vi "XNET Convert (Byte Array to Frame FlexRay).vi"(0 "session in":refnum<k21>, 5 "signal data":u8[](array[numeric]), 11 "error in (no error)":errorcluster) -> (4 "session out":refnum<k21>, 6 "frame data":T1[](array[typedef]) {"payload" format="%x"; "timestamp" format="%<%.7X\n%x>T"; "type" items=["FlexRay Data"=32, "FlexRay Null"=33, "FlexRay Symbol"=34, "Log Trigger"=225, "Start Trigger"=226]; "cycle count" max=63 step=1}, 14 "unused payloads":cluster{"payload":u8[]}[](array[cluster]), 15 "error out":errorcluster)   [LabVIEW 2018]
doc: "Converts signal data to NI-XNET FlexRay frame data."
uses:
  XNET Frame FlexRay.ctl
  XNET Frame Type FlexRay.ctl
  nixlvapi.dll
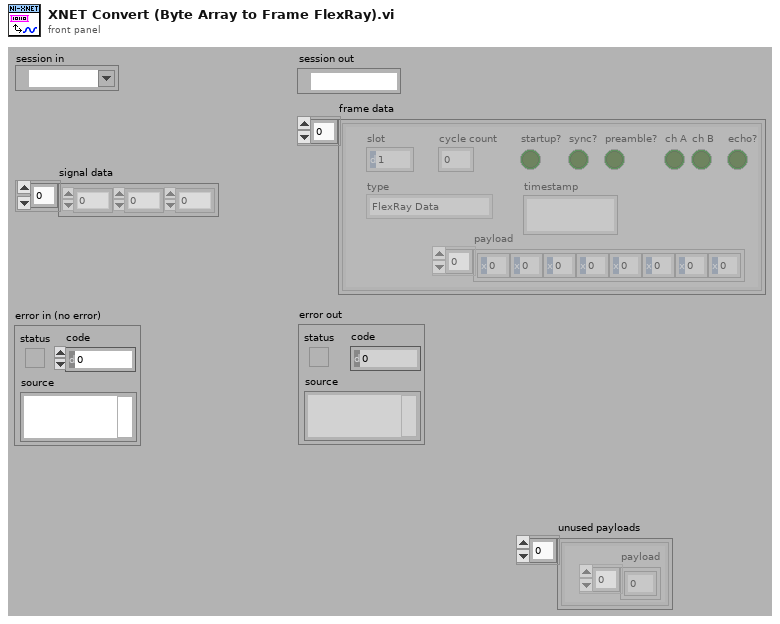
[diagram p1: front panel]
types:
  T1 = typedef "XNET Frame FlexRay.ctl" = cluster{"timestamp":timestamp, "payload":u8[], "slot":u16, "type":T2, "cycle count":u8, "startup?":bool, "sync?":bool, "preamble?":bool, "ch A":bool, "ch B":bool, "echo?":bool}
  T2 = typedef "XNET Frame Type FlexRay.ctl" = u8
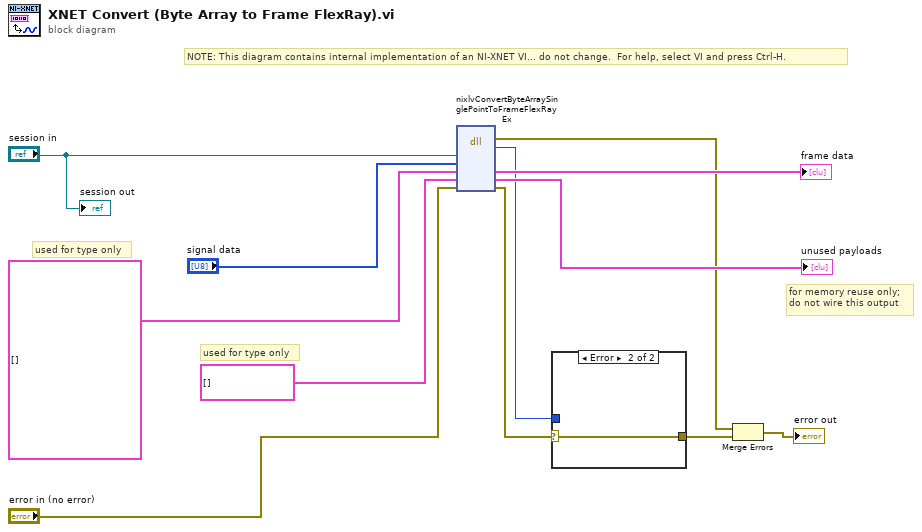
[diagram p0: block diagram]
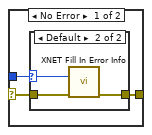
[diagram p2: hidden frame]
diagram:
  # "used for type only"
  # "for memory reuse only;\ndo not wire this output"
  # "used for type only"
  # "NOTE: This diagram contains internal implementation of an NI-XNET VI... do not change.  For help, select VI and press Ctrl-H."
  n1 = dll-call lib="nixlvapi.*" fn="nixlvConvertByteArraySinglePointToFrameFlexRayEx" ("Call Library")("sessionRef"="session in", "signalData"="signal data", "frameData"=T1[] [] ("data"), "unusedPayloads"=cluster{"payload":u8[]}[] [] ("payload array"), "errorInOut"="error in (no error)") -> (error out=w1:errorcluster, "return type"=w4:i32, "frameData"=→"frame data":T1[], "unusedPayloads"=→"unused payloads":cluster{"payload":u8[]}[], "errorInOut"=w3:errorcluster)  [unwired: 4 in, 2 out]
  n2 = case shown="Error" w3 {
    selector: w3 -> [w13 w20]
    tunnel: [w15 w20] -> w12
    tunnel: w4 -> [w14 _]
    frame No Error {
      n3 = case shown="Default" w14 {
        selector: w14 -> [_ w17]
        tunnel: w13 -> [w16 w18]
        tunnel: [w16 w19] -> w15
        frame 0 {
        }
        frame Default {
          n4 = call "XNET Fill In Error Info.vi"("status code"=w17, "error in"=w18) -> ("error out"=w19:errorcluster)  [unwired: 13 out]
        }
      }
    }
    frame Error {
    }
  }
  n5 = Merge Errors(w1, w12) -> (→"error out":errorcluster)
  "session out" <- "session in"
